vi "AI test Drive Relays All v6.vi"(9 "Array #2":bool[](array[boolean]), 10 "Array #1":bool[](array[boolean]), 11 "Array #0":bool[](array[boolean])) -> (0 "error Array":errorcluster[](array[cluster]))   [LabVIEW 2013]
panel:
  in  "stop":bool
  # "LAB01-1 (START)"
  # "LAB02-1 (JIG)"
  # "LAB04-2 (START)"
  # "LAB01-1 (JIG)"
  # "LAB03-1 (START)"
  # "LAB04-2 (JIG)"
  # "LAB01-2 (START)"
  # "LAB05-1 (START)"
  # "LAB03-1 (JIG)"
  # "LAB01-2 (JIG)"
  # "LAB05-1 (JIG)"
  # "LAB03-2 (START)"
  # "LAB02-1 (START)"
  # "LAB05-2 (START)"
  # "LAB03-2 (JIG)"
  # "LAB05-2 (JIG)"
  # "LAB02-1 (JIG)"
  # "LAB04-1 (START)"
  # "LAB02-1 (START)"
  # "LAB04-1 (JIG)"
  # "RESET ALL"
  # "RESET TEMP"
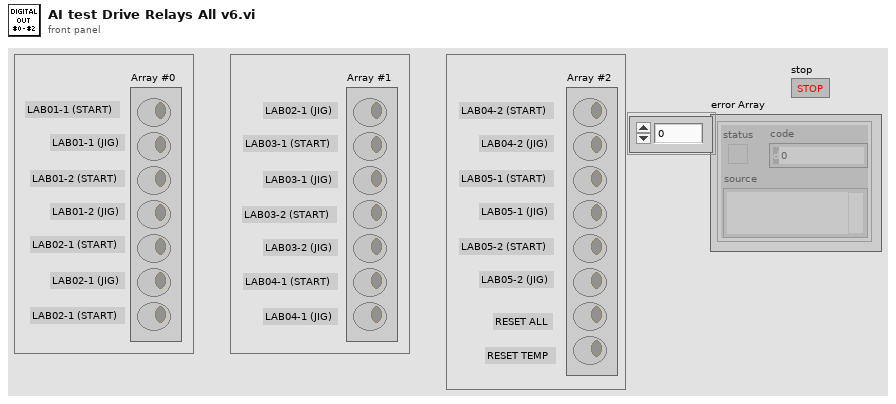
[diagram p1: front panel]
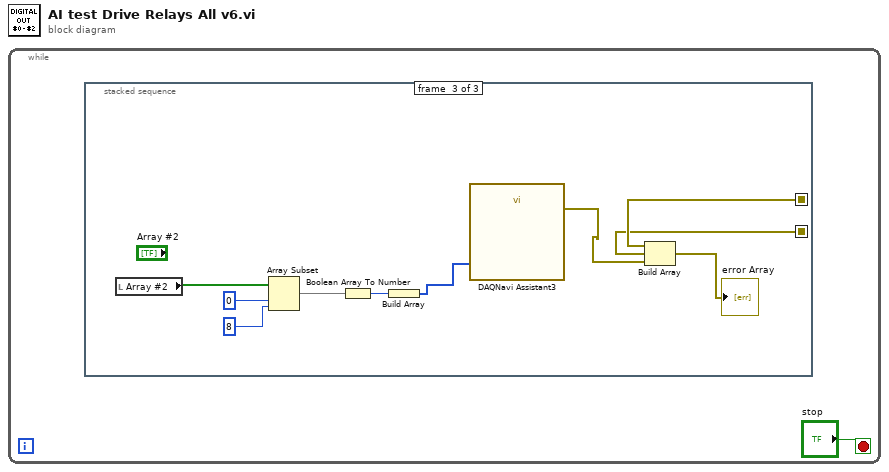
[diagram p0: block diagram]
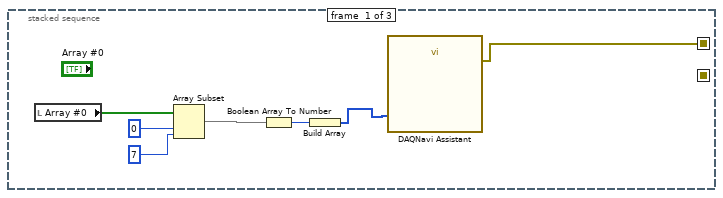
[diagram p2: hidden frame]
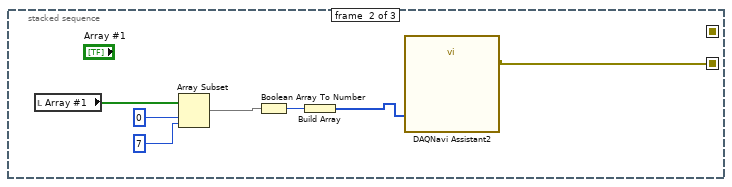
[diagram p3: hidden frame]
diagram:
  n1 = while {
    stop <- "stop" stop-if-true
    n2 = stacked-sequence {
      seq-local: [w2 _ _] -> [_ _ w20]
      seq-local: [_ w9 _] -> [_ _ w19]
      frame #0 {
        n3 = local read "Array #0"() -> (w7:bool[])
        n4 = Array Subset(array=w7, index=0, length=7) -> (w4:bool[])
        n5 = Boolean Array To Number(Boolean array=w4) -> (number=w8:u8)
        n6 = Build Array(w8) -> (w3:u8[])
        n7 = call "DAQNavi Assistant"("dataIn(U8Array)"=w3) -> ("error out"=w2:errorcluster)  [unwired: 26 in]
      }
      frame #1 {
        n8 = local read "Array #1"() -> (w12:bool[])
        n9 = Array Subset(array=w12, index=0, length=7) -> (w11:bool[])
        n10 = Boolean Array To Number(Boolean array=w11) -> (number=w15:u8)
        n11 = Build Array(w15) -> (w10:u8[])
        n12 = call "DAQNavi Assistant2"("dataIn(U8Array)"=w10) -> ("error out"=w9:errorcluster)  [unwired: 26 in]
      }
      frame #2 {
        n13 = local read "Array #2"() -> (w22:bool[])
        n14 = Array Subset(array=w22, index=0, length=8) -> (w21:bool[])
        n15 = Boolean Array To Number(Boolean array=w21) -> (number=w25:u8)
        n16 = Build Array(w25) -> (w17:u8[])
        n17 = call "DAQNavi Assistant3"("dataIn(U8Array)"=w17) -> ("error out"=w16:errorcluster)  [unwired: 26 in]
        n18 = Build Array(w20, w19, w16) -> (→"error Array":errorcluster[])
      }
    }
  }
